vi "leftarmfk.vi"() -> ()   [LabVIEW 2017]
uses:
  1ec58f78-5c71-4f4d-92cd-3dcba08cc06a.vi
  f6a98d5d-64e4-49b0-b16f-dda8a964be0f.vi
  global variable.vi
panel:
  out "추가된 배열 2":dbl[](array[numeric])
  out "newed 2":dbl
  out "left arm distance":dbl
  in  "정지":bool
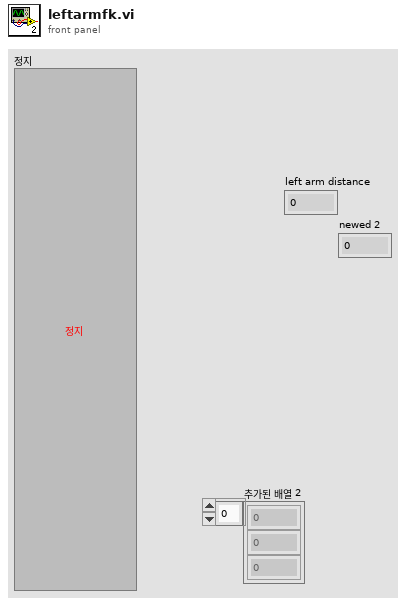
[diagram p1: front panel]
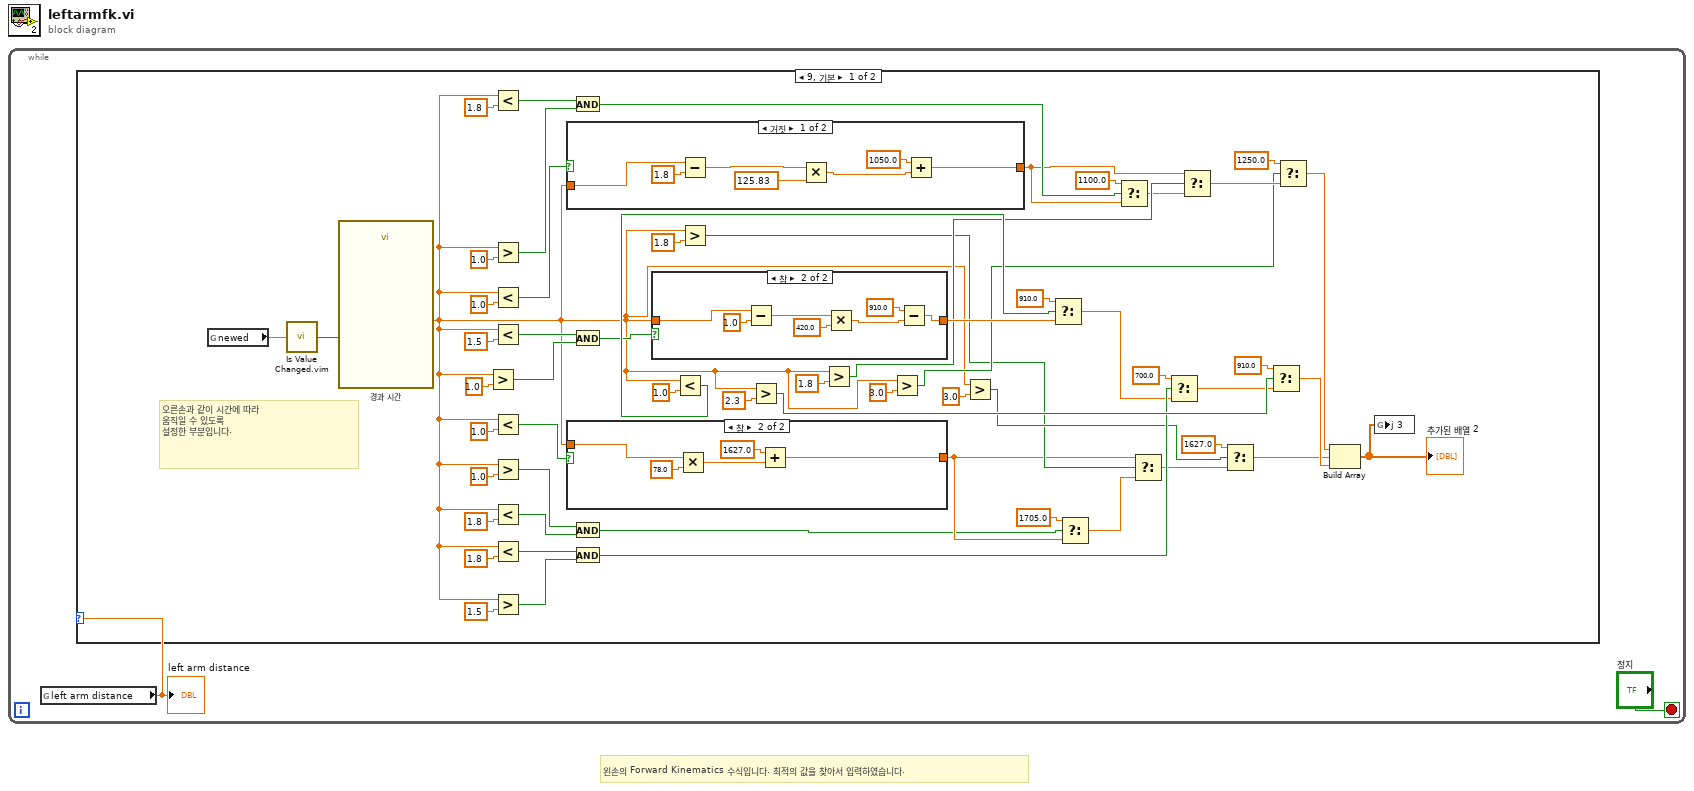
[diagram p0: block diagram]
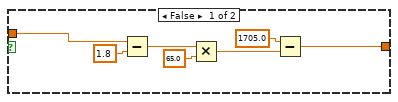
[diagram p2: hidden frame]
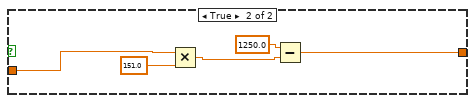
[diagram p3: hidden frame]
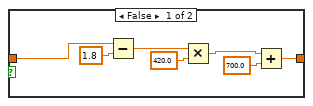
[diagram p4: hidden frame]
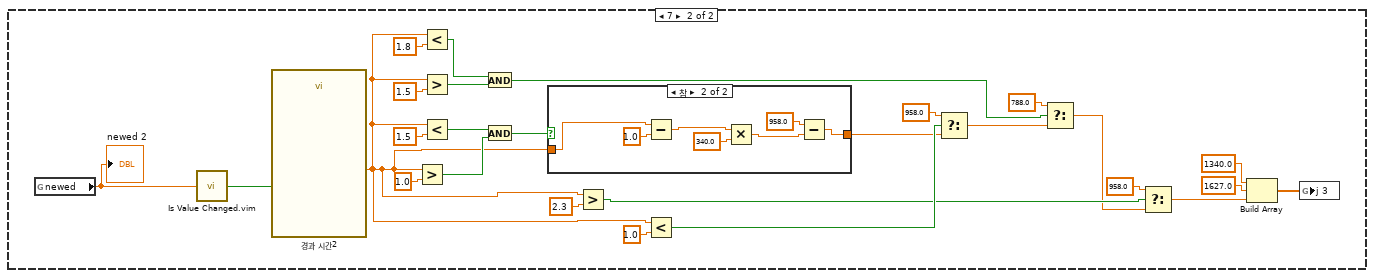
[diagram p5: hidden frame]
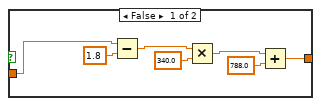
[diagram p6: hidden frame]
diagram:
  # "왼손의 Forward Kinematics 수식입니다. 최적의 값을 찾아서 입력하였습니다."
  n1 = while {
    stop <- "정지" stop-if-true
    n2 = global read "global variable.vi" "left arm distance"() -> (w1:dbl)
    "left arm distance" <- w1
    n3 = case shown="9, 기본" w1 {
      frame 9, Default {
        # "오른손과 같이 시간에 따라\n움직일 수 있도록\n설정한 부분입니다."
        n4 = global read "global variable.vi" "newed"() -> (w4:dbl)
        n5 = call "Is Value Changed.vim"("value"=w4) -> ("changed or first call?"=w61:bool)
        n6 = call "경과 시간"("Reset"=w61) -> ("Elapsed Time (s)"=w7:dbl)  [unwired: 11 in, 7 out]
        n7 = Greater?(x=w7, y=1.0) -> (0:w55:bool)
        n8 = Less?(x=w7, y=1.8) -> (x < y?=w34:bool)
        n9 = Greater?(x=w7, y=1.0) -> (0:w35:bool)
        n10 = Less?(x=w7, y=1.0) -> (x < y?=w29:bool)
        n11 = Less?(x=w7, y=1.5) -> (x < y?=w54:bool)
        n12 = Less?(x=w7, y=1.0) -> (x < y?=w5:bool)
        n13 = Greater?(x=w7, y=1.0) -> (0:w9:bool)
        n14 = Less?(x=w7, y=1.8) -> (x < y?=w10:bool)
        n15 = Less?(x=w7, y=1.8) -> (x < y?=w49:bool)
        n16 = Greater?(x=w7, y=1.5) -> (0:w50:bool)
        n17 = case shown="거짓" w29 {
          tunnel: w7 -> [w77 w81]
          tunnel: [w74 w84] -> w28
          frame False {
            n18 = Subtract(x=w77, y=1.8) -> (x-y=w78:dbl)
            n19 = Multiply(x=w78, y=125.83) -> (x*y=w75:dbl)
            n20 = Add(x=1050.0 ("y"), y=w75) -> (x+y=w74:dbl)
          }
          frame True {
            n21 = Multiply(x=w81, y=151.0) -> (x*y=w82:dbl)
            n22 = Subtract(x=1250.0, y=w82) -> (x-y=w84:dbl)
          }
        }
        n23 = case shown="참" w5 {
          tunnel: w7 -> [w65 w69]
          tunnel: [w62 w72] -> w13
          frame False {
            n24 = Subtract(x=w65, y=1.8) -> (x-y=w66:dbl)
            n25 = Multiply(x=w66, y=65.0) -> (x*y=w63:dbl)
            n26 = Subtract(x=1705.0 ("y"), y=w63) -> (x-y=w62:dbl)
          }
          frame True {
            n27 = Multiply(x=w69, y=78.0) -> (x*y=w70:dbl)
            n28 = Add(x=1627.0, y=w70) -> (x+y=w72:dbl)
          }
        }
        n29 = And(x=w34, y=w35) -> (x .and. y?=w33:bool)
        n30 = And(x=w54, y=w55) -> (x .and. y?=w45:bool)
        n31 = And(x=w9, y=w10) -> (x .and. y?=w8:bool)
        n32 = And(x=w49, y=w50) -> (x .and. y?=w44:bool)
        n33 = case shown="참" w45 {
          tunnel: w7 -> [w86 w95]
          tunnel: [w89 w98] -> w40
          frame False {
            n34 = Subtract(x=w86, y=1.8) -> (x-y=w87:dbl)
            n35 = Multiply(x=w87, y=420.0) -> (x*y=w92:dbl)
            n36 = Add(x=w92, y=700.0) -> (x+y=w89:dbl)
          }
          frame True {
            n37 = Subtract(x=w95, y=1.0) -> (x-y=w93:dbl)
            n38 = Multiply(x=w93, y=420.0) -> (x*y=w96:dbl)
            n39 = Subtract(x=910.0, y=w96) -> (x-y=w98:dbl)
          }
        }
        n40 = Less?(x=w7, y=1.0) -> (x < y?=w59:bool)
        n41 = Greater?(x=w7, y=1.8) -> (0:w14:bool)
        n42 = Greater?(x=w7, y=2.3) -> (0:w48:bool)
        n43 = Greater?(x=w7, y=1.8) -> (0:w38:bool)
        n44 = Greater?(x=w7, y=3.0) -> (0:w25:bool)
        n45 = Greater?(x=w7, y=3.0) -> (0:w18:bool)
        n46 = Select(t=910.0, s=w59, f=w40) -> (s? t:f=w41:dbl)
        n47 = Select(t=1705.0, s=w8, f=w13) -> (s? t:f=w17:dbl)
        n48 = Select(t=1100.0, s=w33, f=w28) -> (s? t:f=w31:dbl)
        n49 = Select(t=w13, s=w14, f=w17) -> (s? t:f=w20:dbl)
        n50 = Select(t=700.0, s=w44, f=w41) -> (s? t:f=w42:dbl)
        n51 = Select(t=w28, s=w38, f=w31) -> (s? t:f=w26:dbl)
        n52 = Select(t=1627.0, s=w18, f=w20) -> (s? t:f=w21:dbl)
        n53 = Select(t=910.0, s=w48, f=w42) -> (s? t:f=w46:dbl)
        n54 = Select(t=1250.0, s=w25, f=w26) -> (s? t:f=w23:dbl)
        n55 = Build Array(w23, w21, w46) -> (w3:dbl[])
        "추가된 배열 2" <- w3
        n56 = global write "global variable.vi" "j 3"(w3) -> ()
      }
      frame 7 {
        n57 = global read "global variable.vi" "newed"() -> (w100:dbl)
        "newed 2" <- w100
        n58 = call "Is Value Changed.vim"("value"=w100) -> ("changed or first call?"=w126:bool)
        n59 = call "경과 시간2"("Reset"=w126) -> ("Elapsed Time (s)"=w102:dbl)  [unwired: 11 in, 7 out]
        n60 = Greater?(x=w102, y=1.0) -> (0:w118:bool)
        n61 = Less?(x=w102, y=1.8) -> (x < y?=w112:bool)
        n62 = Greater?(x=w102, y=1.5) -> (0:w113:bool)
        n63 = Less?(x=w102, y=1.5) -> (x < y?=w117:bool)
        n64 = And(x=w112, y=w113) -> (x .and. y?=w107:bool)
        n65 = And(x=w117, y=w118) -> (x .and. y?=w108:bool)
        n66 = case shown="참" w108 {
          tunnel: w102 -> [w127 w136]
          tunnel: [w130 w139] -> w103
          frame False {
            n67 = Subtract(x=w127, y=1.8) -> (x-y=w128:dbl)
            n68 = Multiply(x=w128, y=340.0) -> (x*y=w133:dbl)
            n69 = Add(x=w133, y=788.0) -> (x+y=w130:dbl)
          }
          frame True {
            n70 = Subtract(x=w136, y=1.0) -> (x-y=w134:dbl)
            n71 = Multiply(x=w134, y=340.0) -> (x*y=w137:dbl)
            n72 = Subtract(x=958.0, y=w137) -> (x-y=w139:dbl)
          }
        }
        n73 = Greater?(x=w102, y=2.3) -> (0:w111:bool)
        n74 = Less?(x=w102, y=1.0) -> (x < y?=w122:bool)
        n75 = Select(t=958.0, s=w122, f=w103) -> (s? t:f=w104:dbl)
        n76 = Select(t=788.0, s=w107, f=w104) -> (s? t:f=w105:dbl)
        n77 = Select(t=958.0, s=w111, f=w105) -> (s? t:f=w109:dbl)
        n78 = Build Array(1340.0 ("원소"), 1627.0 ("원소"), w109) -> (w101:dbl[])
        n79 = global write "global variable.vi" "j 3"(w101) -> ()
      }
    }
  }
